vi "WebView2 Droplet.vi"() -> ()   [LabVIEW 2020, in "WebView2 QControl.lvlib"]
uses:
  WebView2 QControl.lvlib
  C:/Users/Simon/Documents/GitHub/LV-WebView2/Source/Libs/Microsoft.Web.WebView2.WinForms.dll
  Libs/Microsoft.Web.WebView2.WinForms.dll
  WebView2 QControl/WebView2 QControl.lvclass/WebView2 QControl.ctl
  WebView2 QControl/Write URL.vi
  Webview2 Lib/WebView2 Control Object/Write URL.vi
  WebView2 QControl/WebView2 QControl.lvclass
panel:
  in  "WebView2":refnum<k24>(container)
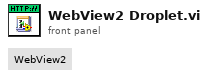
[diagram p1: front panel]
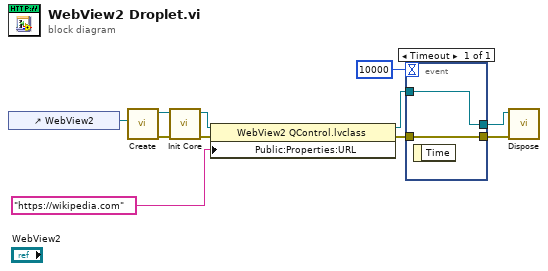
[diagram p0: block diagram]
diagram:
  n1 = control-ref of="WebView2"() -> (w4:refnum<vi>)
  n2 = call "Create.vi"("WebView2 Control Ref"=w4) -> ("error out"=w11:errorcluster, "WebView2 Control out"=w9:refnum<class "WebView2 QControl.lvclass">)  [unwired: 9 in]
  n3 = call "Init Core.vi"("error in (no error)"=w11, "WebView2 Control in"=w9) -> ("error out"=w10:errorcluster, "WebView2 Control out"=w2:refnum<class "WebView2 QControl.lvclass">)  [unwired: 8 in]
  n4 = property class="WebView2 QControl.lvclass"(reference=w2, error in=w10, "Public:Properties:URL"="https://wikipedia.com" ("uri")) -> (reference out=w8:refnum<class "WebView2 QControl.lvclass">, error out=w6:errorcluster)
  n5 = event shown="[0] Timeout" {
    selector: _ -> [_]
    dyn-events: _ -> [_]
    timeout: 10000 -> [_]
    tunnel: [w13] -> w3
    tunnel: w8 -> [w13]
    tunnel: [w12] -> w7
    tunnel: w6 -> [w12]
    event Timeout {
      n6 = event-data() -> ()  [unwired: 1 in, 1 out]
    }
  }
  n7 = call "Dispose.vi"("error in (no error)"=w7, "WebView2 Control in"=w3) -> ()  [unwired: 9 in, 1 out]
